vi "Scaler.vi"(7 "Array1":dbl[](array[numeric]), 11 "Array2":dbl[](array[numeric])) -> (3 "Array_out":dbl[](array[numeric]))   [LabVIEW 2014]
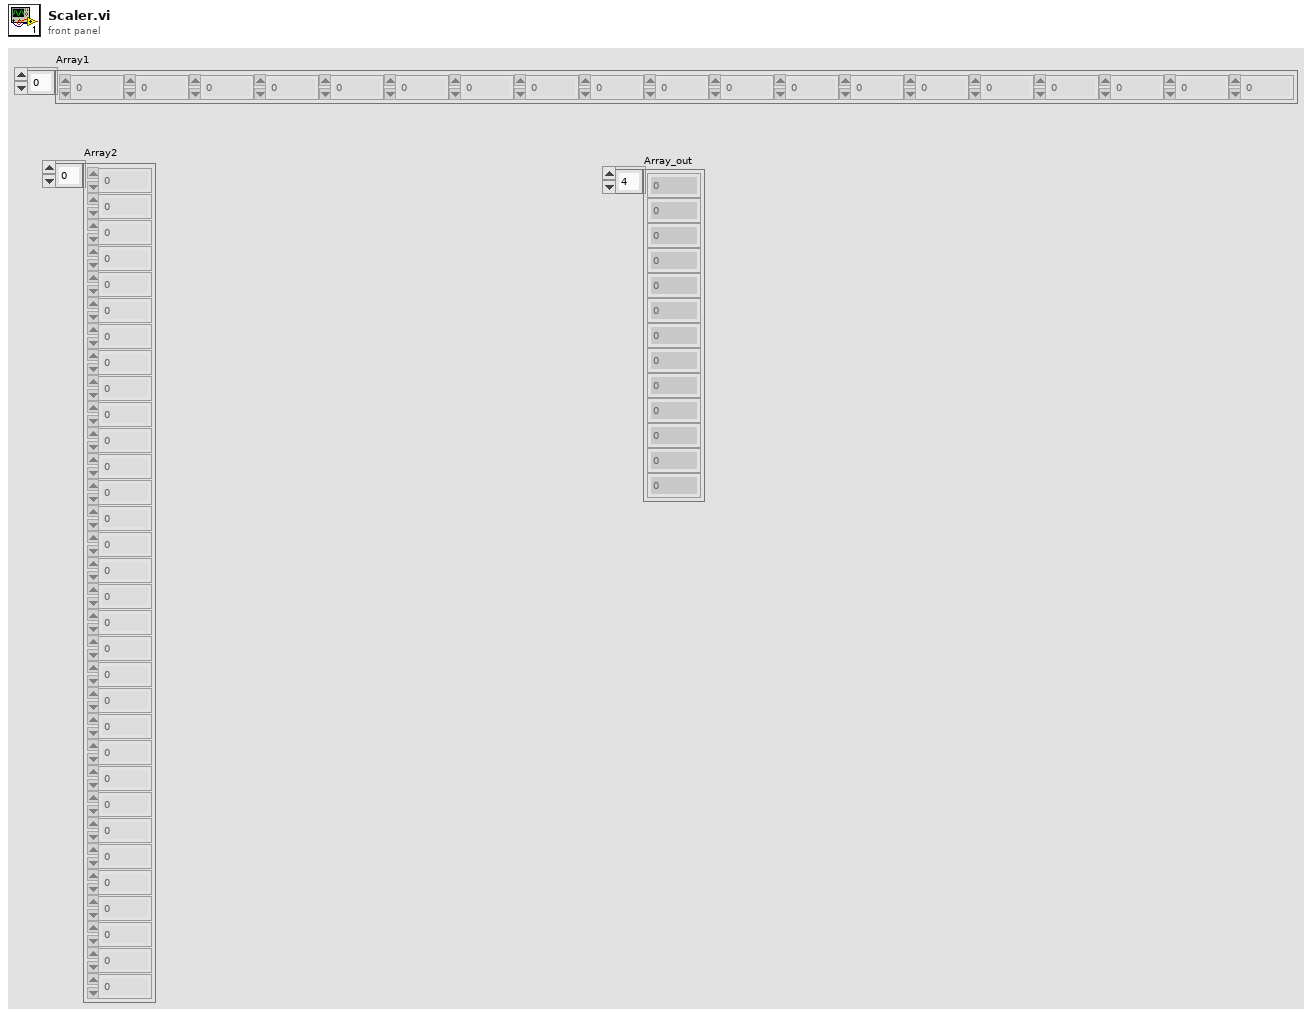
[diagram p1: front panel]
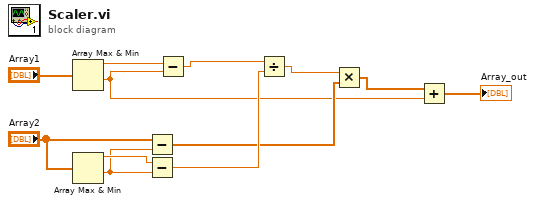
[diagram p0: block diagram]
diagram:
  n1 = Array Max & Min(array="Array1") -> (max value=w9:dbl, min value=w2:dbl)  [unwired: 2 out]
  n2 = Array Max & Min(array="Array2") -> (max value=w10:dbl, min value=w3:dbl)  [unwired: 2 out]
  n3 = Subtract(x="Array2", y=w3) -> (x-y=w5:dbl[])
  n4 = Subtract(x=w10, y=w3) -> (x-y=w7:dbl)
  n5 = Subtract(x=w9, y=w2) -> (x-y=w8:dbl)
  n6 = Divide(x=w8, y=w7) -> (x/y=w6:dbl)
  n7 = Multiply(x=w6, y=w5) -> (x*y=w4:dbl[])
  n8 = Add(x=w4, y=w2) -> (x+y=→"Array_out":dbl[])
